vi "Test Set Row Values Error.vi"(11 "Test Case In":refnum<class "Test Open Xml.lvclass">) -> (0 "error out":errorcluster, 3 "Test Case Out":refnum<class "Test Open Xml.lvclass">)   [LabVIEW 2020, in "Test Open Xml.lvclass"]
uses:
  Test Open Xml.lvclass
  <vilib>/Astemes/LUnit/Test Case.lvclass
  Source/Open Xml.lvlib
  Source/Cell DataType.ctl
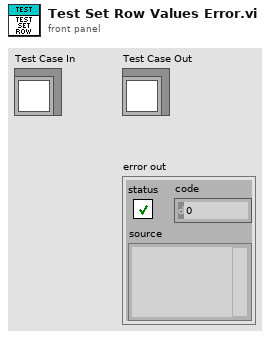
[diagram p1: front panel]
types:
  T1 = typedef "Open Xml.lvlib/Cell DataType.ctl" = enum16{"Void", "Boolean", "Number", "Error", "SharedString", "String", "InlineString", "Date"}
  T2 = cluster{"Number":dbl, "String":string, "Boolean":bool, "Time Stamp":timestamp, "Error":errorcluster}[]
  T3 = cluster{"Number":dbl, "String":string, "Boolean":bool, "Time Stamp":timestamp, "Error":errorcluster}
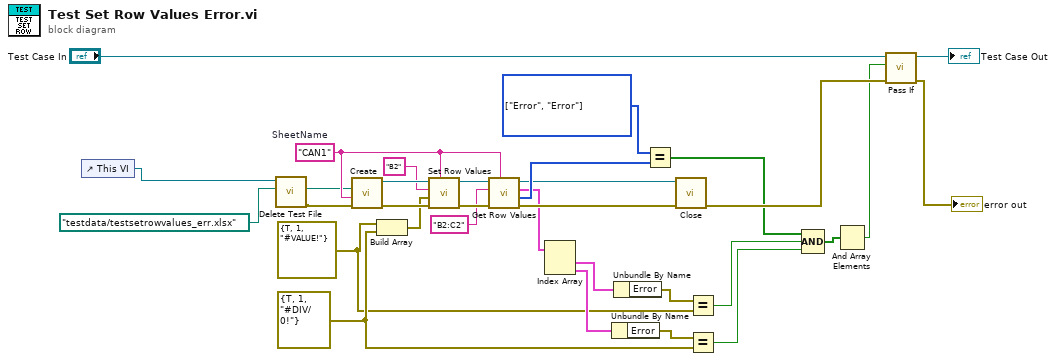
[diagram p0: block diagram]
diagram:
  w5 = errorcluster {"status"=TRUE, "code"=1, "source"="#VALUE!"} ("error constant")
  w6 = errorcluster {"status"=TRUE, "code"=1, "source"="#DIV/0!"} ("error constant")
  w17 = T1[] [enum."Error", enum."Error"] items=["Void", "Boolean", "Number", "Error", "SharedString", "String", "InlineString", "Date"] ("x")
  w7 = "CAN1"  # SheetName
  n1 = control-ref of="This VI"() -> (w2:refnum<vi>)
  n2 = call "Delete Test File.vi"("name or relative path"=path "testdata/testsetrowvalues_err.xlsx", "VI in"=w2) -> ("error out"=w4:errorcluster, "deleted path"=w3:path)  [unwired: 8 in]
  n3 = call "Create.vi"("error in"=w4, "SheetName"=w7, "Path"=w3) -> ("error out"=w28:errorcluster, "SpreadsheetDoc"=w29:refnum<k24>)  [unwired: 7 in]
  n4 = Build Array(w5, w6) -> (w12:errorcluster[])
  n5 = call "Set Row Values.vi"("Sheet Name"=w7, "error in"=w28, "Values"=w12, "Cell Address"="B2", "SpreadsheetDoc"=w29) -> ("error out"=w24:errorcluster, "SpreadsheetDoc out"=w23:refnum<k24>)  [unwired: 5 in]
  n6 = call "Get Row Values.vi"("Sheet Name"=w7, "error in"=w24, "Cell Addresses"="B2:C2" ("Cell Address"), "SpreadsheetDoc in"=w23) -> ("error out"=w26:errorcluster, "Types"=w22:T1[], "Cell Values"=w18:T2, "SpreadsheetDoc out"=w8:refnum<k24>)  [unwired: 4 in]
  n7 = Index Array(array=w18) -> (element #1=w16:T3, element #2=w15:T3)  [unwired: 2 in]
  n8 = Unbundle By Name(w15) -> ("Error"=w10:errorcluster)
  n9 = Unbundle By Name(w16) -> ("Error"=w13:errorcluster)
  n10 = Equal?(x=w17, y=w22) -> (x = y?=w21:bool[])
  n11 = call "Close.vi"("error in"=w26, "SpreadsheetDoc"=w8) -> ("error out"=w27:errorcluster)  [unwired: 9 in]
  n12 = Equal?(x=w13, y=w5) -> (x = y?=w9:bool)
  n13 = Equal?(x=w10, y=w6) -> (x = y?=w11:bool)
  n14 = Compound Arithmetic op=AND(w21, w9, w11) -> (w14:bool[])
  n15 = And Array Elements(Boolean array=w14) -> (logical AND=w25:bool)
  n16 = call <vilib>:"Pass If.vi"("error in (no error)"=w27, "Pass?"=w25, "LUnit Test Case In"="Test Case In") -> ("error out"=→"error out":errorcluster, "LUnit Test Case Out"=→"Test Case Out":refnum<class "Test Open Xml.lvclass">)  [unwired: 7 in]
